vi "Cluster1.vi"() -> ()   [LabVIEW 2020]
panel:
  out "mensaje2":string
  out "Numero2":i32
  out "Cluster":T1={"Numero1"=0, "Numero2"=0, "Numero3"=0, "mensaje1"="", "mensaje2"="", "mensaje3"="", "bool1"=TRUE, "bool2"=TRUE, "bool3"=TRUE}
  in  "Stop Button":bool
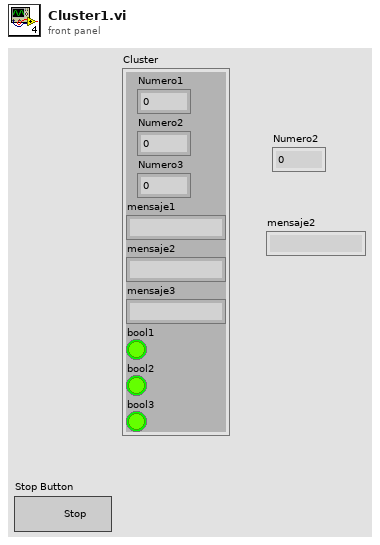
[diagram p1: front panel]
types:
  T1 = cluster{"Numero1":i32, "Numero2":i32, "Numero3":i32, "mensaje1":string, "mensaje2":string, "mensaje3":string, "bool1":bool, "bool2":bool, "bool3":bool}
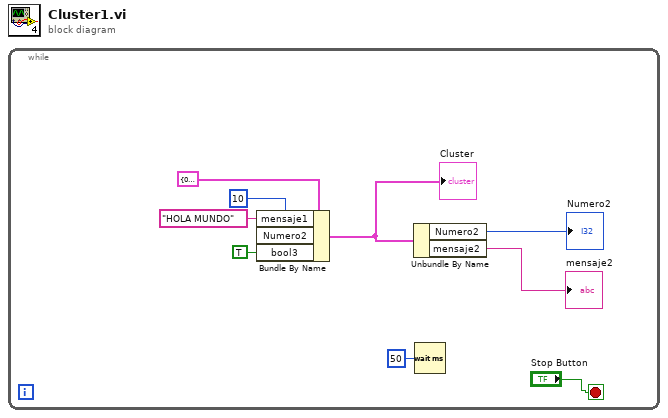
[diagram p0: block diagram]
diagram:
  n1 = while {
    stop <- "Stop Button" stop-if-true
    n2 = Bundle By Name(cluster=T1 {"Numero1"=0, "Numero2"=12, "Numero3"=0, "mensaje1"="", "mensaje2"="", "mensaje3"="", "bool1"=FALSE, "bool2"=FALSE, "bool3"=FALSE}, "mensaje1"="HOLA MUNDO", "Numero2"=10, "bool3"=TRUE) -> (w4:T1)
    "Cluster" <- w4
    n3 = Unbundle By Name(w4) -> ("Numero2"=→"Numero2":i32, "mensaje2"=→"mensaje2":string)
    n4 = Wait (ms)(milliseconds to wait=u32 50) -> ()  [unwired: 1 out]
  }
